vi "Screen label master.vi"() -> ()   [LabVIEW 2017]
uses:
  <vilib>/Utility/error.llb/DialogType.ctl
  <vilib>/Utility/file.llb/Read From Spreadsheet File (string).vi
  <vilib>/Utility/file.llb/Write To Spreadsheet File (string).vi
panel:
  out "error out":errorcluster
  in  "error in (no error)":errorcluster
  in  "Exit":bool
  in  "Save":bool
  in  "Screen Names":T1
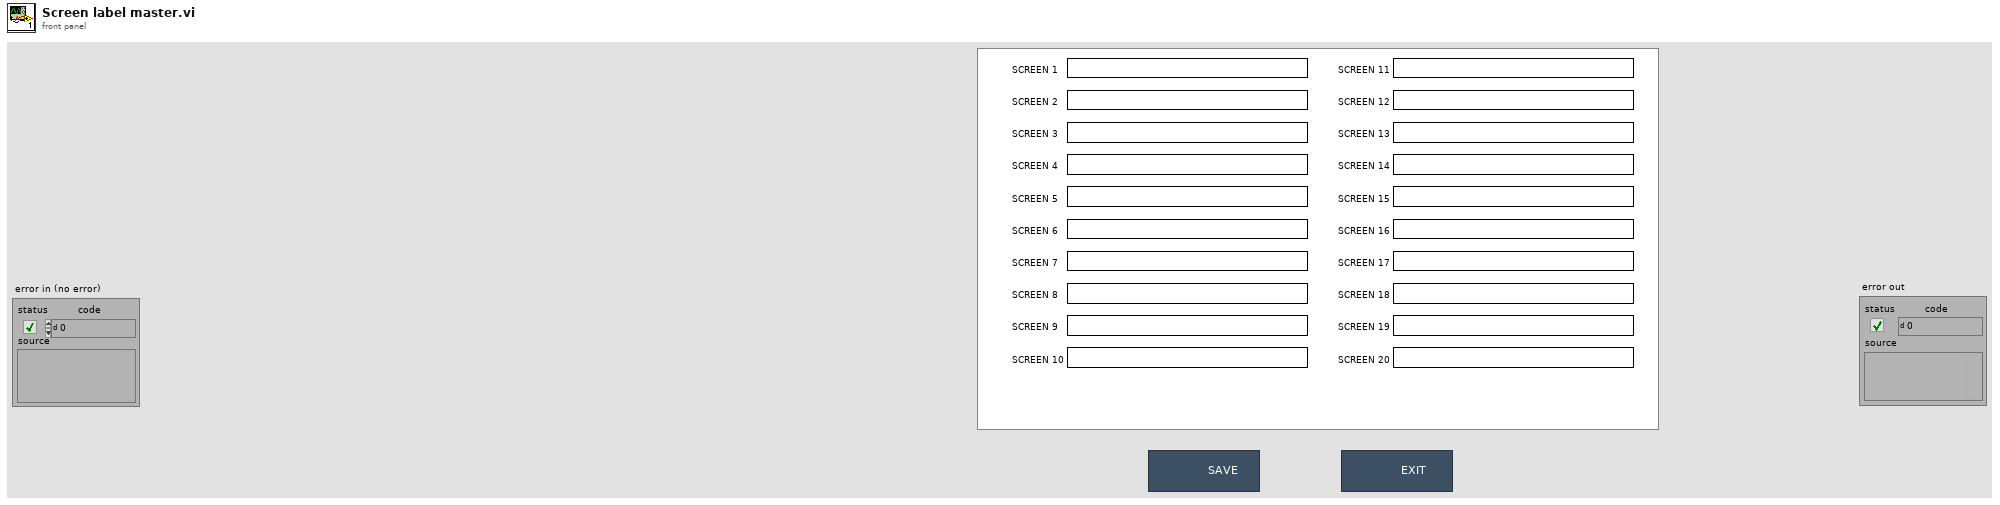
[diagram p1: front panel]
types:
  T1 = cluster{"SCREEN 1":string, "SCREEN 2":string, "SCREEN 3":string, "SCREEN 4":string, "SCREEN 5":string, "SCREEN 6":string, "SCREEN 7":string, "SCREEN 8":string, "SCREEN 9":string, "SCREEN 10":string, "SCREEN 11":string, "SCREEN 12":string, "SCREEN 13":string, "SCREEN 14":string, "SCREEN 15":string, "SCREEN 16":string, "SCREEN 17":string, "SCREEN 18":string, "SCREEN 19":string, "SCREEN 20":string}
  T2 = typedef "DialogType.ctl" = u16
  T3 = enum32{"invalid app kind", "Development System", "Run Time System", "Student Edition", "Embedded LabVIEW", "Evaluation", "Custom"}
  T4 = cluster{"first row[0]":string, "first row[1]":string, "first row[2]":string, "first row[3]":string, "first row[4]":string, "first row[5]":string, "first row[6]":string, "first row[7]":string, "first row[8]":string, "first row[9]":string, "first row[10]":string, "first row[11]":string, "first row[12]":string, "first row[13]":string, "first row[14]":string, "first row[15]":string, "first row[16]":string, "first row[17]":string, "first row[18]":string, "first row[19]":string}
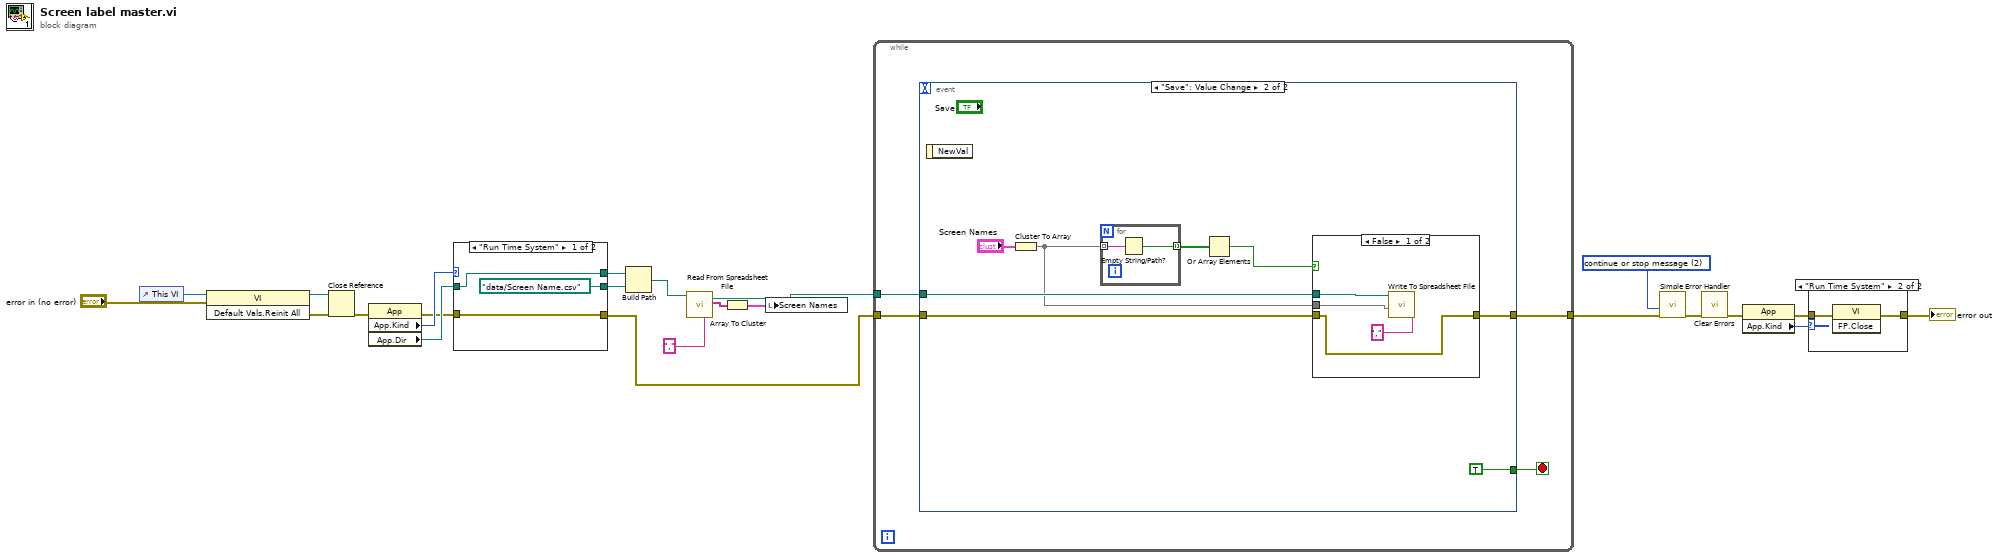
[diagram p0: block diagram]
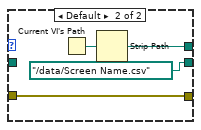
[diagram p3: hidden frame]
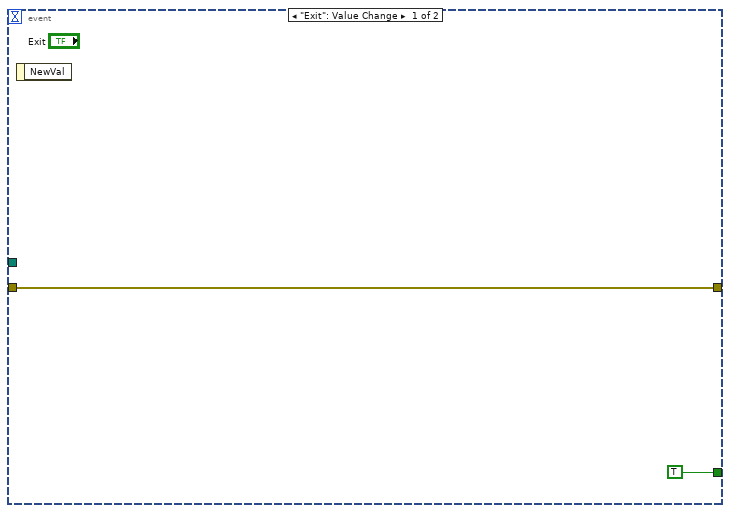
[diagram p4: hidden frame]
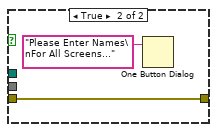
[diagram p5: hidden frame]
diagram:
  w4 = T2 2 items=["no dialog", "OK message", "continue or stop message", "OK message + warnings", "continue/stop + warnings"] ("type of dialog (OK msg:1)")
  n1 = control-ref of="This VI"() -> (w23:refnum<vi>)
  n2 = invoke class="VI" method="Default Vals.Reinit All"(reference=w23, error in="error in (no error)") -> (reference out=w20:refnum<vi>, error out=w21:errorcluster)  [unwired: 1 in, 1 out]
  n3 = Close Reference(reference=w20, error in (no error)=w21) -> (error out=w17:errorcluster)
  n4 = property class="App"(error in=w17) -> (error out=w16:errorcluster, "App.Kind"=w19:T3, "App.Dir"=w18:path)  [unwired: 1 in, 1 out]
  n5 = case shown="\"Run Time System\"" w19 {
    tunnel: w18 -> [w26 _]
    tunnel: [path "data/Screen Name.csv" ("path") path "../data/Screen Name.csv" ("path")] -> w15
    tunnel: [w26 w28] -> w14
    tunnel: w16 -> [w24 w27]
    tunnel: [w24 w27] -> w2
    frame "Run Time System" {
    }
    frame Default {
      n6 = Current VI's Path() -> (path=w29:path)
      n7 = Strip Path(path=w29) -> (stripped path=w28:path)  [unwired: 1 out]
    }
  }
  n8 = Build Path(base path=w14, name or relative path=w15) -> (appended path=w13:path)
  n9 = call-poly <vilib>:"Read From Spreadsheet File.vi"("delimiter (\\t)"="," ("delimiter (\\t)"), "file path (dialog if empty)"=w13) -> ("first row"=w1:string[], "new file path (Not A Path if cancelled)"=w12:path)  [unwired: 5 in, 3 out]
  n10 = Array To Cluster(array=w1) -> (cluster=w10:T4)
  n11 = local write "Screen Names"(w10) -> ()
  n12 = while {
    tunnel: w2 -> [w34]
    tunnel: w12 -> [w32]
    tunnel: [w31] -> w3
    stop <- w33 stop-if-true
    n13 = event shown="[1] \"Save\": Value Change" {
      selector: _ -> [_ _]
      dyn-events: _ -> [_ _]
      timeout: _ -> [_ _]
      tunnel: w34 -> [w36 w42]
      tunnel: [w36 w41] -> w31
      tunnel: [TRUE TRUE] -> w33
      tunnel: w32 -> [_ w40]
      event "Exit": Value Change {
        n14 = event-data() -> ()  [unwired: 1 in, 1 out]
      }
      event "Save": Value Change {
        n15 = event-data() -> ()  [unwired: 1 in, 1 out]
        n16 = Cluster To Array(cluster="Screen Names") -> (array=w39:string[])
        n17 = for {
          tunnel: w39 -> [w46] mode=indexing
          tunnel: [w45] -> w38 mode=indexing
          n18 = Empty String/Path?(string/path=w46) -> (empty?=w45:bool)
        }
        n19 = Or Array Elements(Boolean array=w38) -> (logical OR=w37:bool)
        n20 = case shown="False" w37 {
          tunnel: w42 -> [w48 w52]
          tunnel: [w48 w52] -> w41
          tunnel: w40 -> [w50 _]
          tunnel: w39 -> [w47 _]
          frame False {
            n21 = call-poly <vilib>:"Write To Spreadsheet File.vi"("delimiter (\\t)"="," ("delimiter (\\t)"), "1D data"=w47, "file path (dialog if empty)"=w50) -> ()  [unwired: 5 in, 1 out]
          }
          frame True {
            n22 = One Button Dialog(message="Please Enter Names\nFor All Screens...") -> ()  [unwired: 1 in, 1 out]
          }
        }
      }
    }
  }
  n23 = call <vilib>:"Simple Error Handler.vi"("type of dialog (OK msg:1)"=w4, "error in (no error)"=w3) -> ("error out"=w9:errorcluster)  [unwired: 3 in, 4 out]
  n24 = call <vilib>:"Clear Errors.vi"("error in (no error)"=w9) -> ("error out"=w6:errorcluster)  [unwired: 5 in, 1 out]
  n25 = property class="App"(error in=w6) -> (error out=w7:errorcluster, "App.Kind"=w8:T3)  [unwired: 1 in, 1 out]
  n26 = case shown="\"Run Time System\"" w8 {
    tunnel: w7 -> [w53 w55]
    tunnel: [w53 w54] -> w5
    frame Default {
    }
    frame "Run Time System" {
      n27 = invoke class="VI" method="FP.Close"(error in=w55) -> (error out=w54:errorcluster)  [unwired: 2 in, 2 out]
    }
  }
  "error out" <- w5
